vi "GetTreeChilds.vi"(9 "Tag":string, 10 "error in (no error)":errorcluster, 11 "Tree Refnum":refnum<vi>) -> (1 "Childs":string[](array[string]), 2 "error out":errorcluster, 3 "Tree Refnum":refnum<vi>)   [LabVIEW 2021, in "Tree.lvlib" / "Tree.lvclass"]
uses:
  Tree.lvclass
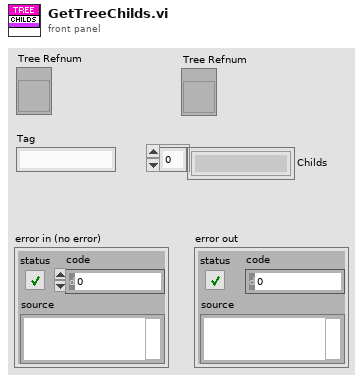
[diagram p1: front panel]
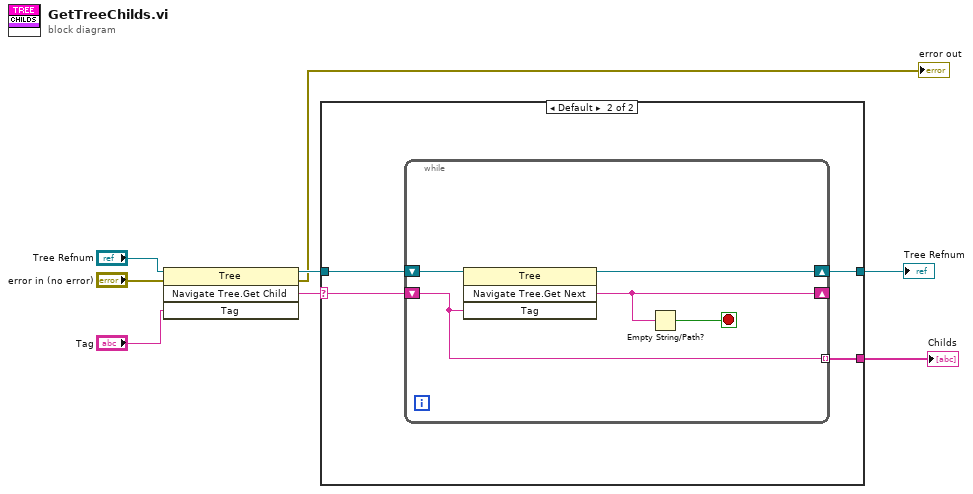
[diagram p0: block diagram]
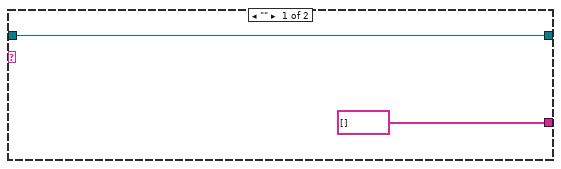
[diagram p2: hidden frame]
diagram:
  n1 = invoke class="Tree" method="Navigate Tree.Get Child"(reference="Tree Refnum", error in="error in (no error)", "Tag"="Tag") -> (reference out=w5:refnum<vi>, error out=→"error out":errorcluster, "Navigate Tree:Get Child"=w4:string)  [unwired: 1 in, 1 out]
  n2 = case shown="Default" w4 {
    selector: w4 -> [_ w12]
    tunnel: [w10 w14] -> w8
    tunnel: w5 -> [w10 w13]
    tunnel: [string[] [] ("Childs") w11] -> w2
    frame "" {
    }
    frame Default {
      n3 = while {
        shift-right: [w18] -> w14
        shift-left: w13 -> [w19]
        shift-right: [w16] -> _
        shift-left: w12 -> [w17]
        tunnel: [w17] -> w11 mode=indexing
        stop <- w15 stop-if-true
        n4 = invoke class="Tree" method="Navigate Tree.Get Next"(reference=w19, "Tag"=w17) -> (reference out=w18:refnum<vi>, "Navigate Tree:Get Next Item"=w16:string)  [unwired: 2 in, 2 out]
        n5 = Empty String/Path?(string/path=w16) -> (empty?=w15:bool)
      }
    }
  }
  "Tree Refnum" <- w8
  "Childs" <- w2
